vi "LV_multiports_multiservers.vi"() -> ()   [LabVIEW 2020]
panel:
  out "2nd port":string
  out "1st port":string
  in  "Open Multi Ports":bool
  in  "Send Test Image":bool
  in  "h":i32=10 min=1 max=5000 step=1
  in  "w":i32=1 min=1 max=5000 step=1
  out "Elaps ms":u32
  in  "Send Image":bool
  out "Path to Python script":path
  in  "Stop":bool
  out "Answer":string
  in  "Ping":bool
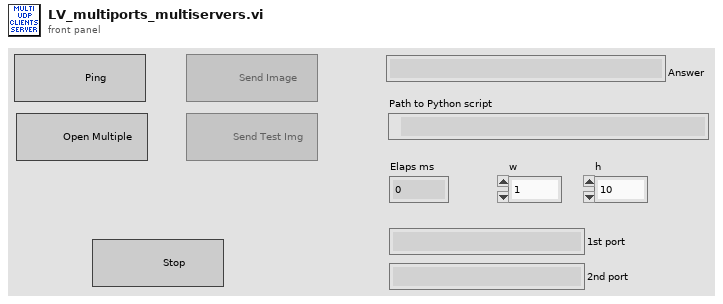
[diagram p1: front panel]
types:
  T1 = enum8{"Enabled", "Disabled", "Disabled and Grayed Out"}
  T2 = typedef "Image Type" = u32
  T3 = typedef "IMAQ Image.ctl" = refnum<image>
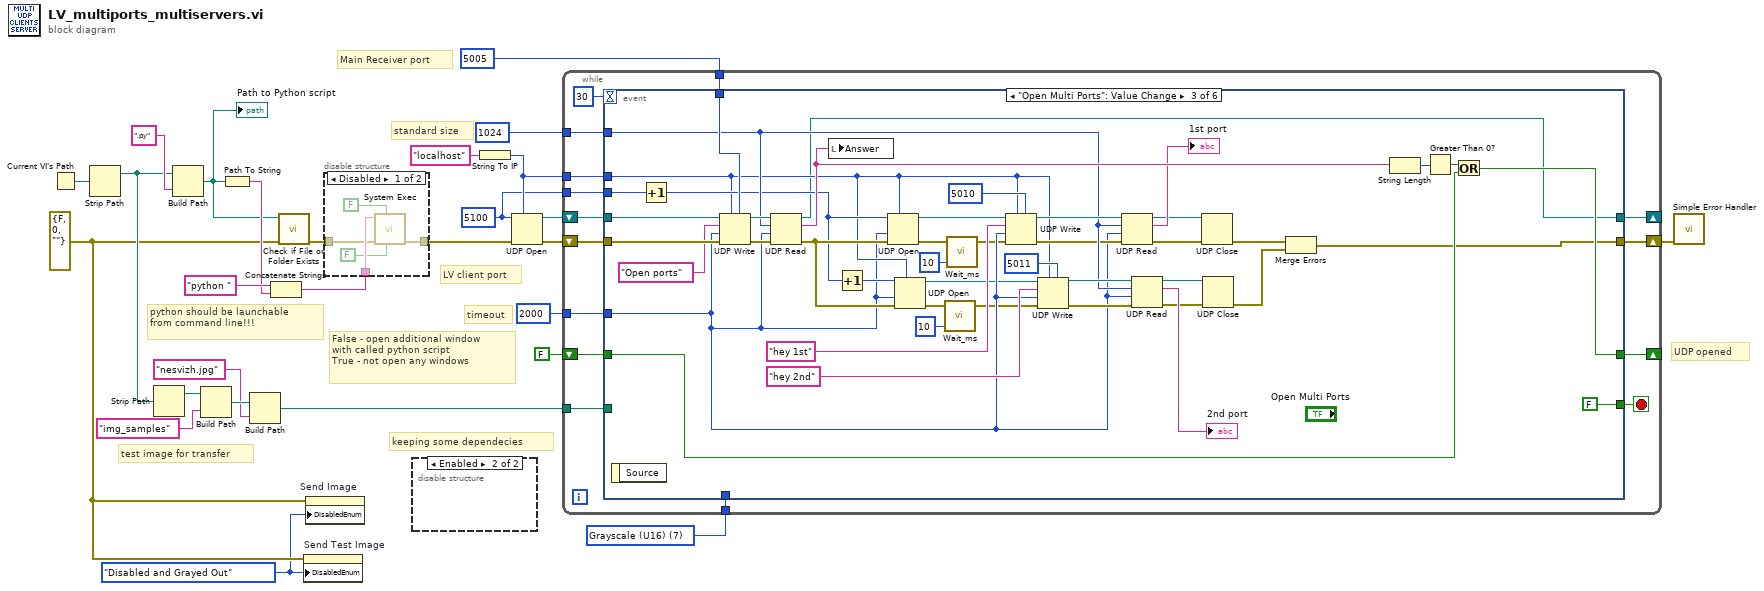
[diagram p0: block diagram]
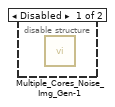
[diagram p2: hidden frame]
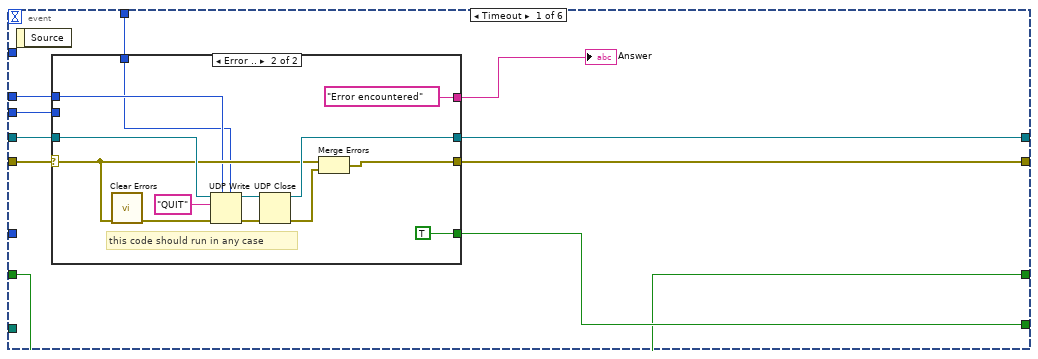
[diagram p4: hidden frame]
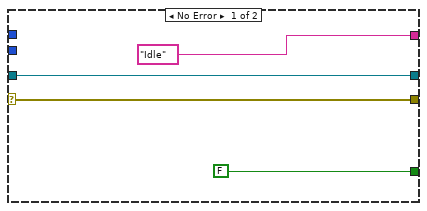
[diagram p5: hidden frame]
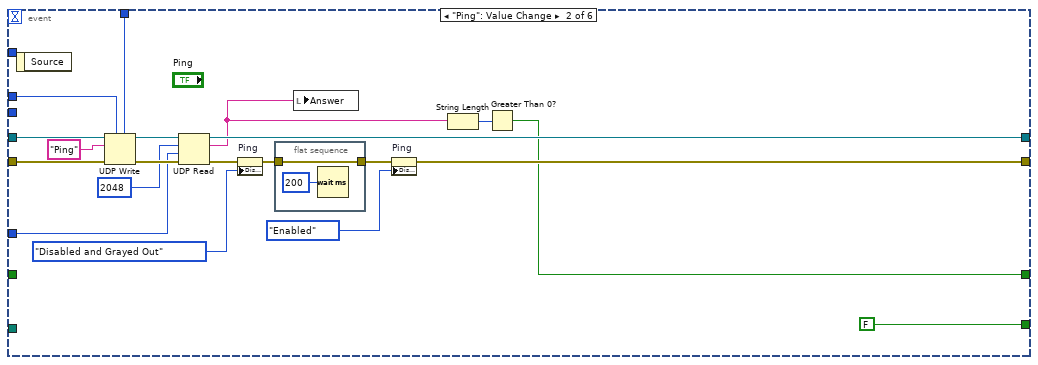
[diagram p6: hidden frame]
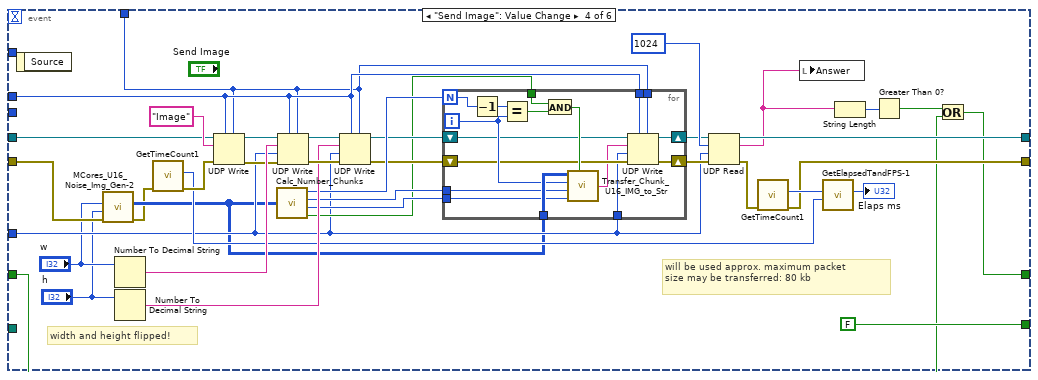
[diagram p7: hidden frame]
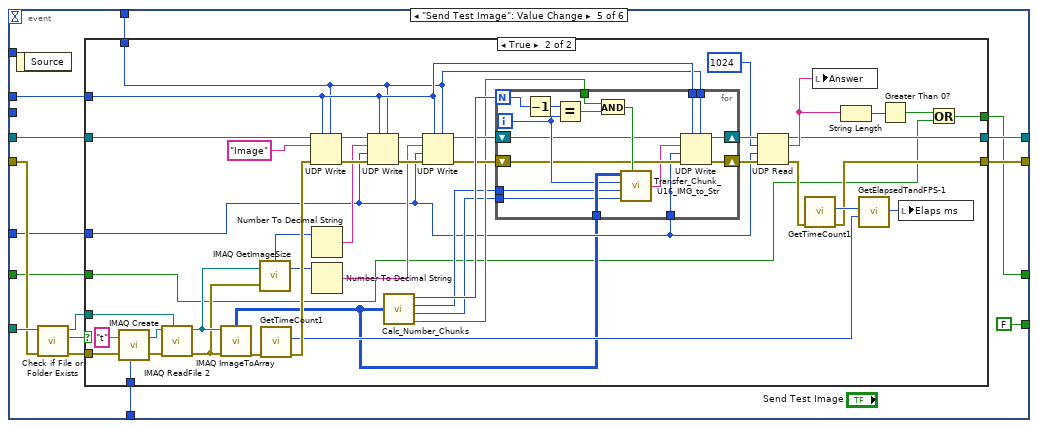
[diagram p8: hidden frame]
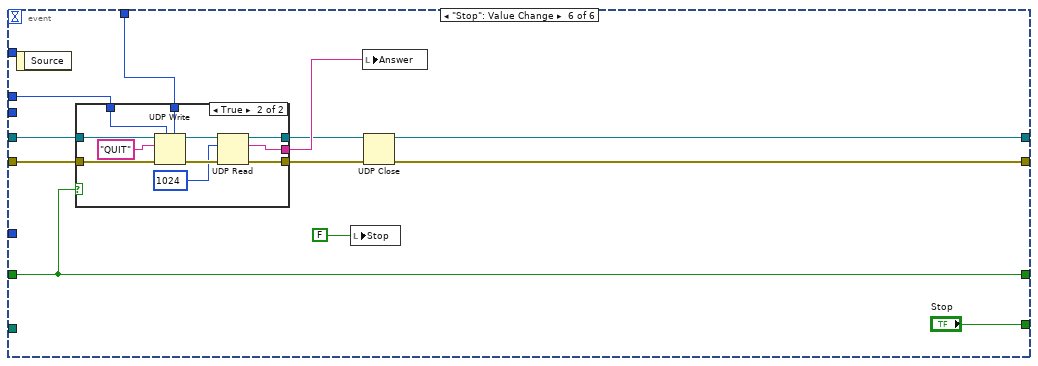
[diagram p10: hidden frame]
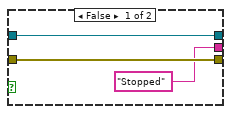
[diagram p11: hidden frame]
diagram:
  w3 = T1."Disabled and Grayed Out" ("Disabled")
  w5 = T2 7 items=["Grayscale (U8)", "Grayscale (I16)", "Grayscale (SGL)", "Complex (CSG)", "RGB (U32)", "HSL (U32)", "RGB (U64)", "Grayscale (U16)"] ("Image Type")
  w14 = u16 5100 ("remote port or service name")
  w4 = errorcluster {"status"=FALSE, "code"=0, "source"=""} ("error in (no error)")
  # "standard size"
  # "UDP opened"
  # "test image for transfer"
  # "keeping some dependecies"
  # "timeout"
  # "Main Receiver port"
  # "LV client port"
  # "False - open additional window\nwith called python script\nTrue - not open any windows"
  # "python should be launchable \nfrom command line!!!"
  n1 = Current VI's Path() -> (path=w26:path)
  n2 = Strip Path(path=w26) -> (stripped path=w11:path)  [unwired: 1 out]
  n3 = Strip Path(path=w11) -> (stripped path=w10:path)  [unwired: 1 out]
  n4 = Build Path(base path=w11, name or relative path=".py" ("string")) -> (appended path=w21:path)
  "Path to Python script" <- w21
  n5 = Build Path(base path=w10, name or relative path="img_samples" ("string")) -> (appended path=w8:path)
  n6 = Path To String(path=w21) -> (string=w22:string)
  n7 = Build Path(base path=w8, name or relative path="nesvizh.jpg" ("string")) -> (appended path=w6:path)
  n8 = Concatenate Strings("python " ("command line"), w22) -> (w24:string)
  n9 = call <vilib>:"Check if File or Folder Exists.vi"("error in (no error)"=w4, "path"=w21) -> ("error out"=w20:errorcluster)  [unwired: 7 in, 2 out]
  n10 = property on="Send Test Image" class="Bool"(error in=w4, "DisabledEnum"=w3) -> ()  [unwired: 1 in, 2 out]
  n11 = property on="Send Image" class="Bool"(error in=w4, "DisabledEnum"=w3) -> ()  [unwired: 1 in, 2 out]
  n12 = disable-structure shown="Disabled" {
    disable-tunnel: w24 -> [w32 _]
    disable-tunnel: [w31 w33] -> w19
    disable-tunnel: w20 -> [w29 w33]
    frame Disabled {
      n13 = call <vilib>:"System Exec.vi"("run minimized? (F)"=FALSE, "wait until completion? (T)"=FALSE, "error in (no error)"=w29, "command line"=w32) -> ("error out"=w31:errorcluster)  [unwired: 4 in, 3 out]
    }
    frame Enabled {
    }
  }
  n14 = disable-structure shown="Enabled" {
    frame Disabled {
      n15 = call "Multiple_Cores_Noise_Img_Gen-1.vi"() -> ()  [unwired: 10 in, 2 out]
    }
    frame Enabled {
    }
  }
  n16 = String To IP(1:"localhost" ("address")) -> (0:w15:u32)
  n17 = UDP Open(7:w15, 8:w19, 11:w14) -> (port=w17:refnum<k16>, 0:w18:errorcluster)  [unwired: 2 in, 1 out]
  n18 = while {
    shift-right: [w45] -> _
    shift-left: w17 -> [w46]
    shift-right: [w43] -> w27
    shift-left: w18 -> [w47]
    tunnel: w15 -> [w41]
    tunnel: w14 -> [w42]
    tunnel: u16 5005 ("remote port or service name") -> [w40]
    tunnel: 2000 -> [w39]
    tunnel: w6 -> [w38]
    tunnel: w5 -> [w37]
    shift-right: [w35] -> _
    shift-left: FALSE -> [w36]
    tunnel: 1024 -> [w34]
    stop <- w44 stop-if-true
    n19 = event shown="[2] \"Open Multi Ports\": Value Change" {
      selector: _ -> [_ _ _ _ _ _]
      dyn-events: _ -> [_ _ _ _ _ _]
      timeout: 30 -> [_ _ _ _ _ _]
      tunnel: [w54 FALSE ("Stop") FALSE ("Stop") FALSE ("Stop") FALSE ("Stop") "Stop"] -> w44
      tunnel: w47 -> [w58 w89 w142 w152 w210 w283]
      tunnel: w46 -> [w57 w88 w140 w179 w205 w284]
      tunnel: [w56 w84 w110 w173 w200 w285] -> w45
      tunnel: [w55 w91 w122 w165 w201 w286] -> w43
      tunnel: w42 -> [w52 _ w118 _ _ _]
      tunnel: w41 -> [w51 w81 w113 w154 w204 w279]
      tunnel: w40 -> [w50 w80 w139 w153 w203 w278]
      tunnel: w39 -> [_ w79 w112 w155 w202 _]
      tunnel: w38 -> [_ _ _ _ w211 _]
      tunnel: w37 -> [_ _ _ _ w206 _]
      tunnel: w36 -> [w49 _ w129 w144 w198 w277]
      tunnel: [w49 w76 w128 w143 w199 w277] -> w35
      tunnel: w34 -> [_ _ w125 _ _ _]
      event Timeout {
        n20 = event-data() -> ()  [unwired: 1 in, 1 out]
        n21 = case shown="Error .." w58 {
          selector: w58 -> [w61 w70]
          tunnel: [w62 w73] -> w56
          tunnel: w57 -> [w62 w72]
          tunnel: [w61 w71] -> w55
          tunnel: [FALSE ("Stop") TRUE ("Stop")] -> w54
          tunnel: ["Idle" ("Answer") "Error encountered" ("Answer")] -> w53
          tunnel: w52 -> [_ _]
          tunnel: w51 -> [_ w69]
          tunnel: w50 -> [_ w68]
          frame No Error {
          }
          frame Error {
            # "this code should run in any case"
            n22 = call <vilib>:"Clear Errors.vi"("error in (no error)"=w70) -> ("error out"=w67:errorcluster)  [unwired: 5 in, 1 out]
            n23 = UDP Write(address=w69, port or service name=w68, connection ID=w72, data in="QUIT", 8:w67) -> (error out=w66:errorcluster, 3:w64:refnum<k16>)  [unwired: 1 in]
            n24 = UDP Close(connection ID=w64, 8:w66) -> (connection ID out=w73:refnum<k16>, error out=w63:errorcluster)
            n25 = Merge Errors(w70, w63) -> (w71:errorcluster)
          }
        }
        "Answer" <- w53
      }
      event "Ping": Value Change {
        n26 = event-data() -> ()  [unwired: 1 in, 1 out]
        n27 = UDP Write(address=w81, port or service name=w80, connection ID=w88, data in="Ping", 8:w89) -> (error out=w86:errorcluster, 3:w85:refnum<k16>)  [unwired: 1 in]
        n28 = UDP Read(connection ID=w85, max size (548)=2048 ("bytes to read"), timeout ms (25000)=w79, 8:w86) -> (data out=w78:string, error out=w83:errorcluster, 3:w84:refnum<k16>)  [unwired: 2 out]
        n29 = property on="Ping" class="Bool"(error in=w83, "DisabledEnum"=T1."Disabled and Grayed Out" ("Disabled")) -> (error out=w94:errorcluster)  [unwired: 1 in, 1 out]
        n30 = flat-sequence {
          tunnel: w94 -> [w96]
          tunnel: [w96] -> w92
          frame #0 {
            n31 = Wait (ms)(milliseconds to wait=u32 200) -> ()  [unwired: 1 out]
          }
        }
        n32 = local write "Answer"(w78) -> ()
        n33 = property on="Ping" class="Bool"(error in=w92, "DisabledEnum"=T1."Enabled" ("Disabled")) -> (error out=w91:errorcluster)  [unwired: 1 in, 1 out]
        n34 = String Length(string=w78) -> (length=w77:i32)
        n35 = Greater Than 0?(x=w77) -> (x > 0?=w76:bool)
      }
      event "Open Multi Ports": Value Change {
        n36 = event-data() -> ()  [unwired: 1 in, 1 out]
        n37 = Increment(x=w118) -> (x+1=w115:u16)
        n38 = UDP Write(address=w113, port or service name=w139, connection ID=w140, data in="Open ports", 8:w142, 9:w112) -> (error out=w138:errorcluster, 3:w137:refnum<k16>)
        n39 = UDP Read(connection ID=w137, max size (548)=w125, timeout ms (25000)=w112, 8:w138) -> (data out=w130:string, error out=w116:errorcluster, 3:w110:refnum<k16>)  [unwired: 2 out]
        n40 = local write "Answer"(w130) -> ()
        n41 = Increment(x=w115) -> (x+1=w114:u16)
        n42 = UDP Open(7:w113, 8:w116, 9:w112, 11:w115) -> (port=w117:refnum<k16>, 0:w103:errorcluster)  [unwired: 1 in, 1 out]
        n43 = UDP Open(7:w113, 8:w116, 9:w112, 11:w114) -> (port=w111:refnum<k16>, 0:w100:errorcluster)  [unwired: 1 in, 1 out]
        n44 = call "Wait_ms.vi"("[IN] Suspend ms"=u32 10, "error IN"=w100) -> ("error OUT"=w99:errorcluster)  [unwired: 3 in]
        n45 = call "Wait_ms.vi"("[IN] Suspend ms"=u32 10, "error IN"=w103) -> ("error OUT"=w102:errorcluster)  [unwired: 3 in]
        n46 = UDP Write(address=w113, port or service name=u16 5010, connection ID=w117, data in="hey 1st", 8:w102, 9:w112) -> (error out=w120:errorcluster, 3:w127:refnum<k16>)
        n47 = UDP Write(address=w113, port or service name=u16 5011, connection ID=w111, data in="hey 2nd", 8:w99, 9:w112) -> (error out=w119:errorcluster, 3:w126:refnum<k16>)
        n48 = UDP Read(connection ID=w127, max size (548)=w125, timeout ms (25000)=w112, 8:w120) -> (data out=→"1st port":string, error out=w109:errorcluster, 3:w108:refnum<k16>)  [unwired: 2 out]
        n49 = UDP Read(connection ID=w126, max size (548)=w125, timeout ms (25000)=w112, 8:w119) -> (data out=→"2nd port":string, error out=w106:errorcluster, 3:w107:refnum<k16>)  [unwired: 2 out]
        n50 = UDP Close(connection ID=w108, 8:w109) -> (error out=w105:errorcluster)  [unwired: 1 out]
        n51 = UDP Close(connection ID=w107, 8:w106) -> (error out=w104:errorcluster)  [unwired: 1 out]
        n52 = Merge Errors(w105, w104) -> (w122:errorcluster)
        n53 = String Length(string=w130) -> (length=w132:i32)
        n54 = Greater Than 0?(x=w132) -> (x > 0?=w131:bool)
        n55 = Or(x=w131, y=w129) -> (x .or. y?=w128:bool)
      }
      event "Send Image": Value Change {
        # "width and height flipped!"
        # "will be used approx. maximum packet \nsize may be transferred: 80 kb"
        n56 = event-data() -> ()  [unwired: 1 in, 1 out]
        n57 = call "MCores_U16_Noise_Img_Gen-2.vi"("error IN"=w152, "[IN] Width"="h", "[IN] Height"="w") -> ("error OUT"=w150:errorcluster, "[OUT] U16 Pixel Img"=w151:u16[][])  [unwired: 7 in]
        n58 = Number To Decimal String(number="w") -> (decimal integer string=w175:string)  [unwired: 1 in]
        n59 = Number To Decimal String(number="h") -> (decimal integer string=w172:string)  [unwired: 1 in]
        n60 = call "GetTimeCount1.vi"("error IN"=w150) -> ("error OUT"=w169:errorcluster, "[OUT] Timer Count"=w166:u32)  [unwired: 9 in]
        n61 = UDP Write(address=w154, port or service name=w153, connection ID=w179, data in="Image", 8:w169) -> (error out=w170:errorcluster, 3:w171:refnum<k16>)  [unwired: 1 in]
        n62 = call "Calc_Number_Chunks.vi"("[IN] U16 Pixel Img"=w151) -> ("[OUT] Number of chunks"=w162:i32, "[OUT] # rows single transfer"=w161:i32, "[OUT] # rows last transfer"=w160:i32, "[OUT] Not-equal last transfer"=w156:bool)
        n63 = UDP Write(address=w154, port or service name=w153, connection ID=w171, data in=w175, 8:w170, 9:w155) -> (error out=w178:errorcluster, 3:w177:refnum<k16>)
        n64 = UDP Write(address=w154, port or service name=w153, connection ID=w177, data in=w172, 8:w178, 9:w155) -> (error out=w158:errorcluster, 3:w159:refnum<k16>)
        n65 = for {
          N: w162 -> [w197]
          shift-right: [w187] -> w163
          shift-left: w158 -> [w188]
          tunnel: w151 -> [w195]
          tunnel: w161 -> [w190]
          tunnel: w160 -> [w189]
          shift-right: [w186] -> w157
          shift-left: w159 -> [w185]
          tunnel: w156 -> [w192]
          tunnel: w155 -> [w183]
          tunnel: w154 -> [w182]
          tunnel: w153 -> [w181]
          i -> [w193]
          n66 = Decrement(x=w197) -> (x-1=w196:i32)
          n67 = Equal?(x=w196, y=w193) -> (x = y?=w191:bool)
          n68 = And(x=w192, y=w191) -> (x .and. y?=w194:bool)
          n69 = call "Transfer_Chunk_U16_IMG_to_Str.vi"("[IN] U16 Pixel Img"=w195, "[IN] # of chunk"=w193, "[IN] # rows single transfer"=w190, "[IN] # rows last transfer"=w189, "[IN] Use remained rows"=w194) -> ("[OUT] Converted String"=w184:string)
          n70 = UDP Write(address=w182, port or service name=w181, connection ID=w185, data in=w184, 8:w188, 9:w183) -> (error out=w187:errorcluster, 3:w186:refnum<k16>)
        }
        n71 = UDP Read(connection ID=w157, max size (548)=1024 ("bytes to read"), timeout ms (25000)=w155, 8:w163) -> (data out=w146:string, error out=w168:errorcluster, 3:w173:refnum<k16>)  [unwired: 2 out]
        n72 = call "GetTimeCount1.vi"("error IN"=w168) -> ("error OUT"=w165:errorcluster, "[OUT] Timer Count"=w167:u32)  [unwired: 9 in]
        n73 = local write "Answer"(w146) -> ()
        n74 = call "GetElapsedTandFPS-1.vi"("[IN] Timer Count Before ALL [ms]"=w166, "[IN] Timer Count After ALL [ms]"=w167) -> ("[OUT] Elapsed time [ms]"=→"Elaps ms":u32)  [unwired: 3 in, 2 out]
        n75 = String Length(string=w146) -> (length=w147:i32)
        n76 = Greater Than 0?(x=w147) -> (x > 0?=w145:bool)
        n77 = Or(x=w145, y=w144) -> (x .or. y?=w143:bool)
      }
      event "Send Test Image": Value Change {
        n78 = event-data() -> ()  [unwired: 1 in, 1 out]
        n79 = call <vilib>:"Check if File or Folder Exists.vi"("error in (no error)"=w210, "path"=w211) -> ("error out"=w209:errorcluster, "file or folder exists?"=w208:bool, "dup path"=w207:path)  [unwired: 7 in]
        n80 = case shown="True" w208 {
          tunnel: w209 -> [w214 w259]
          tunnel: w207 -> [_ w254]
          tunnel: w206 -> [_ w258]
          tunnel: w205 -> [w215 w252]
          tunnel: w204 -> [_ w233]
          tunnel: w203 -> [_ w232]
          tunnel: w202 -> [_ w229]
          tunnel: [w214 w223] -> w201
          tunnel: [w215 w218] -> w200
          tunnel: [w213 w217] -> w199
          tunnel: w198 -> [w213 w216]
          frame False {
          }
          frame True {
            n81 = call "IMAQ Create"("Image Name"="t", "Image Type"=w258, "error in (no error)"=w259) -> ("New Image"=w255:T3, "error out"=w256:errorcluster)  [unwired: 2 in]
            n82 = call "IMAQ ReadFile 2"("File Path"=w254, "error in (no error)"=w256, "Image"=w255) -> ("error out"=w248:errorcluster, "Image Out"=w249:T3)  [unwired: 4 in, 3 out]
            n83 = call "IMAQ ImageToArray"("error in (no error)"=w248, "Image"=w249) -> ("error out"=w253:errorcluster, "Image Pixels (U8)"=w222:u8[][])  [unwired: 2 in, 3 out]
            n84 = call "IMAQ GetImageSize"("Image"=w249, "error in (no error)"=w248) -> ("Y Resolution"=w246:i32, "X Resolution"=w247:i32)  [unwired: 2 in, 1 out]
            n85 = call "GetTimeCount1.vi"("error IN"=w253) -> ("error OUT"=w251:errorcluster, "[OUT] Timer Count"=w226:u32)  [unwired: 9 in]
            n86 = UDP Write(address=w233, port or service name=w232, connection ID=w252, data in="Image", 8:w251) -> (error out=w245:errorcluster, 3:w244:refnum<k16>)  [unwired: 1 in]
            n87 = Number To Decimal String(number=w247) -> (decimal integer string=w243:string)  [unwired: 1 in]
            n88 = Number To Decimal String(number=w246) -> (decimal integer string=w240:string)  [unwired: 1 in]
            n89 = UDP Write(address=w233, port or service name=w232, connection ID=w244, data in=w243, 8:w245, 9:w229) -> (error out=w241:errorcluster, 3:w242:refnum<k16>)
            n90 = call "Calc_Number_Chunks.vi"("[IN] U16 Pixel Img"=w222) -> ("[OUT] Number of chunks"=w239:i32, "[OUT] # rows single transfer"=w235:i32, "[OUT] # rows last transfer"=w234:i32, "[OUT] Not-equal last transfer"=w236:bool)
            n91 = UDP Write(address=w233, port or service name=w232, connection ID=w242, data in=w240, 8:w241, 9:w229) -> (error out=w237:errorcluster, 3:w238:refnum<k16>)
            n92 = for {
              N: w239 -> [w276]
              shift-right: [w266] -> w231
              shift-left: w237 -> [w267]
              tunnel: w222 -> [w274]
              tunnel: w235 -> [w269]
              tunnel: w234 -> [w268]
              shift-right: [w265] -> w230
              shift-left: w238 -> [w264]
              tunnel: w236 -> [w271]
              tunnel: w229 -> [w262]
              tunnel: w233 -> [w261]
              tunnel: w232 -> [w260]
              i -> [w272]
              n93 = Decrement(x=w276) -> (x-1=w275:i32)
              n94 = Equal?(x=w275, y=w272) -> (x = y?=w270:bool)
              n95 = And(x=w271, y=w270) -> (x .and. y?=w273:bool)
              n96 = call "Transfer_Chunk_U16_IMG_to_Str.vi"("[IN] U16 Pixel Img"=w274, "[IN] # of chunk"=w272, "[IN] # rows single transfer"=w269, "[IN] # rows last transfer"=w268, "[IN] Use remained rows"=w273) -> ("[OUT] Converted String"=w263:string)
              n97 = UDP Write(address=w261, port or service name=w260, connection ID=w264, data in=w263, 8:w267, 9:w262) -> (error out=w266:errorcluster, 3:w265:refnum<k16>)
            }
            n98 = UDP Read(connection ID=w230, max size (548)=1024 ("bytes to read"), timeout ms (25000)=w229, 8:w231) -> (data out=w220:string, error out=w228:errorcluster, 3:w218:refnum<k16>)  [unwired: 2 out]
            n99 = call "GetTimeCount1.vi"("error IN"=w228) -> ("error OUT"=w223:errorcluster, "[OUT] Timer Count"=w227:u32)  [unwired: 9 in]
            n100 = local write "Answer"(w220) -> ()
            n101 = String Length(string=w220) -> (length=w221:i32)
            n102 = call "GetElapsedTandFPS-1.vi"("[IN] Timer Count Before ALL [ms]"=w226, "[IN] Timer Count After ALL [ms]"=w227) -> ("[OUT] Elapsed time [ms]"=w224:u32)  [unwired: 3 in, 2 out]
            n103 = Greater Than 0?(x=w221) -> (x > 0?=w219:bool)
            n104 = local write "Elaps ms"(w224) -> ()
            n105 = Or(x=w219, y=w216) -> (x .or. y?=w217:bool)
          }
        }
      }
      event "Stop": Value Change {
        n106 = event-data() -> ()  [unwired: 1 in, 1 out]
        n107 = case shown="True" w277 {
          tunnel: w284 -> [w291 w302]
          tunnel: w283 -> [w290 w301]
          tunnel: [w290 w297] -> w282
          tunnel: ["Stopped" ("data out") w296] -> w281
          tunnel: [w291 w295] -> w280
          tunnel: w279 -> [_ w293]
          tunnel: w278 -> [_ w292]
          frame False {
          }
          frame True {
            n108 = UDP Write(address=w293, port or service name=w292, connection ID=w302, data in="QUIT", 8:w301) -> (error out=w298:errorcluster, 3:w299:refnum<k16>)  [unwired: 1 in]
            n109 = UDP Read(connection ID=w299, max size (548)=1024 ("bytes to read"), 8:w298) -> (data out=w296:string, error out=w297:errorcluster, 3:w295:refnum<k16>)  [unwired: 1 in, 2 out]
          }
        }
        n110 = local write "Stop"(FALSE ("Stop")) -> ()
        n111 = local write "Answer"(w281) -> ()
        n112 = UDP Close(connection ID=w280, 8:w282) -> (connection ID out=w285:refnum<k16>, error out=w286:errorcluster)
      }
    }
  }
  n113 = call <vilib>:"Simple Error Handler.vi"("error in (no error)"=w27) -> ()  [unwired: 4 in, 5 out]
